vi "Initialize (Local Device).vi"(0 "devices":refnum<k21>, 7 "reservation access (Read/Write)":i32(ring)=3 items=["None"=0, "Read Only"=1, "Read/Write"=3], 9 "reservation group":string, 11 "error in (no error)":errorcluster, 12 "connect timeout (60 sec)":dbl=60.0) -> (4 "SLSC Interface out":refnum<class "SLSC Driver.lvclass">, 15 "error out":errorcluster)   [LabVIEW 2015, in "SLSC Driver.lvclass"]
uses:
  SLSC Driver.lvclass
  <vilib>/SLSC/SLSC.lvlib
  <vilib>/SLSC/Initialize Session with Devices.vi
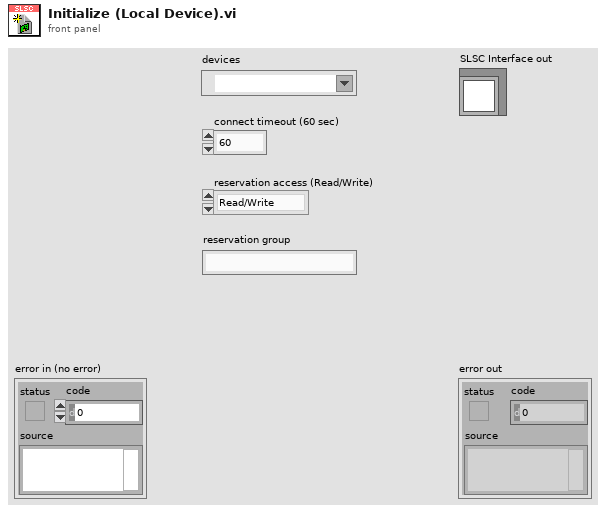
[diagram p1: front panel]
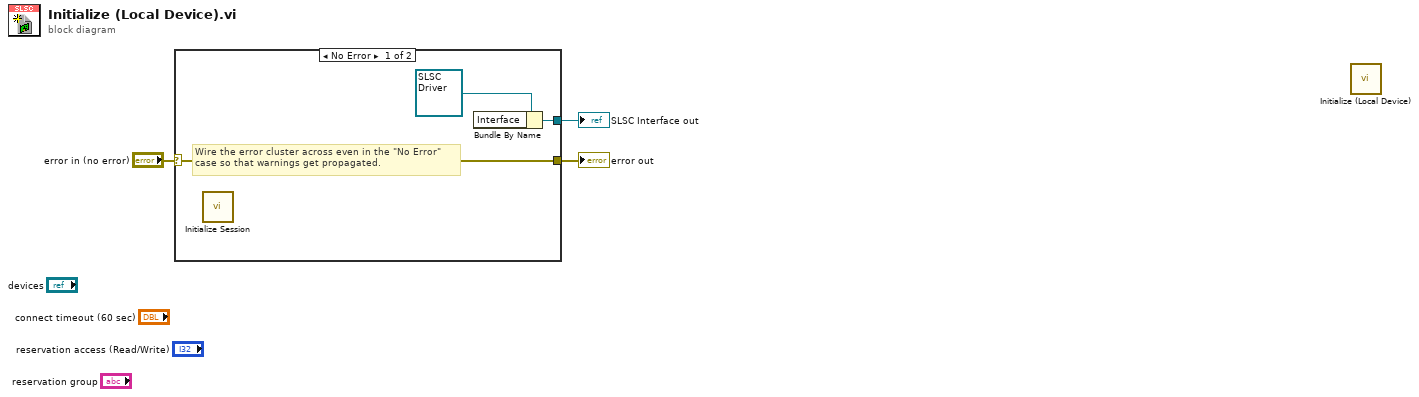
[diagram p0: block diagram]
diagram:
  n1 = case shown="No Error" "error in (no error)" {
    selector: "error in (no error)" -> [w6 w7]
    tunnel: [w6 w7] -> w2
    tunnel: [w4 _] -> w1
    frame No Error {
      # "Wire the error cluster across even in the \"No Error\"\ncase so that warnings get propagated."
      n2 = call-poly <vilib>:"Initialize Session.vi"() -> ()  [unwired: 14 in, 2 out]
      n3 = Bundle By Name(cluster=refnum<class "SLSC Driver.lvclass"> refnum ("SLSC Interface out")) -> (w4:refnum<class "SLSC Driver.lvclass">)  [unwired: 1 in]
    }
    frame Error {
    }
  }
  "error out" <- w2
  "SLSC Interface out" <- w1
  n4 = call "Initialize (Local Device).vi"() -> ()  [unwired: 14 in, 2 out]
